vi "Radians to Degrees (Scalar SGL).vi"(3 "angle (rad)":sgl) -> (1 "angle (deg)":sgl)   [LabVIEW 2017, in "NI_AngleManipulation.lvlib"]
doc: "Converts an angle from radians to degrees."
uses:
  <vilib>/Utility/AngleManip/NI_AngleManipulation.lvlib
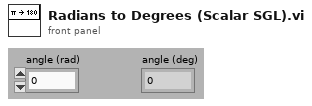
[diagram p1: front panel]
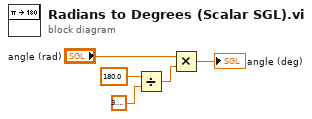
[diagram p0: block diagram]
diagram:
  n1 = Divide(x=sgl 180.0 ("y"), y=sgl 3.1415927) -> (x/y=w2:sgl)
  n2 = Multiply(x="angle (rad)", y=w2) -> (x*y=→"angle (deg)":sgl)
